vi "Persistence.vi"() -> ()   [LabVIEW 2022 SP3]
uses:
  ColorSelection.ctl
  d94e0766-a9f8-4b91-b199-a4dd9911b6b9.vi
  <vilib>/measure/NI_MABase.lvlib
  ed4c178f-8d92-4741-ab18-05d4051c7f8b.vi
panel:
  out "2nd Palette":u32[](array[colorbox])=[16711680, 16715535, 16719390, 16723245, 16727100, 16730955, 16734810, 16738665, 16742520, 16746375, 16750230, 16754085, 16757940, 16761795, 16765650, 16769505, 16773360]
  in  "2ndColor":T1
  in  "Buffer Depth IN":i32=17
  in  "1stColor":T1=enum."Green"
  out "1st Palette":u32[](array[colorbox])=[65280, 1048335, 2031390, 3014445, 3997500, 4980555, 5963610, 6946665, 7929720, 8912775, 9895830, 10878885, 11861940, 12844995, 13828050, 14811105, 15794160]
  in  "Color 2":T1
  in  "Color 1":T1=enum."Green"
  out "Palette 2":u32[](array[colorbox])=[16711680, 16715535, 16719390, 16723245, 16727100, 16730955, 16734810, 16738665, 16742520, 16746375, 16750230, 16754085, 16757940, 16761795, 16765650, 16769505, 16773360]
  in  "Signal Type 2":enum16{"Sine", "Gauss", "Sine + Gauss"}(ring)=enum."Sine + Gauss"
  out "Buffer Depth 2":i32=17
  out "Buffer Depth 1":i32=17
  in  "Combine signals to Signal 2":enum16{"None", "Add 1 and 2"}(ring)
  in  "Signal Type 1":enum16{"Sine", "Gauss", "Sine + Gauss"}(ring)=enum."Sine + Gauss"
  in  "frequency 2":dbl=3.0 format="%0.2p"
  in  "amplitude 2":dbl=0.75 format="%0.2p"
  in  "phase 2 [deg]":dbl=-2.0
  in  "sampling info 2":cluster{"Fs":dbl, "#s":dbl}={"Fs"=1000.0, "#s"=1000.0} {"Fs" format="%.2p"}
  out "Palette 1":u32[](array[colorbox])=[65280, 1048335, 2031390, 3014445, 3997500, 4980555, 5963610, 6946665, 7929720, 8912775, 9895830, 10878885, 11861940, 12844995, 13828050, 14811105, 15794160]
  in  "Persistence Depth":u32=17
  out "Combined Plots":waveform(dbl)[](graph)=[{"t0"=timestamp(0 s since 1904-01-01), "dt"=0.001, "Y"=array[1000 elements]}, {"t0"=timestamp(0 s since 1904-01-01), "dt"=0.001, "Y"=array[1000 elements]}, {"t0"=timestamp(0 s since 1904-01-01), "dt"=0.001, "Y"=array[1000 elements]}, {"t0"=timestamp(0 s since 1904-01-01), "dt"=0.001, "Y"=array[1000 elements]}, {"t0"=timestamp(0 s since 1904-01-01), "dt"=0.001, "Y"=array[1000 elements]}, {"t0"=timestamp(0 s since 1904-01-01), "dt"=0.001, "Y"=array[1000 elements]}, {"t0"=timestamp(0 s since 1904-01-01), "dt"=0.001, "Y"=array[1000 elements]}, {"t0"=timestamp(0 s since 1904-01-01), "dt"=0.001, "Y"=array[1000 elements]}, {"t0"=timestamp(0 s since 1904-01-01), "dt"=0.001, "Y"=array[1000 elements]}, {"t0"=timestamp(0 s since 1904-01-01), "dt"=0.001, "Y"=array[1000 elements]}, {"t0"=timestamp(0 s since 1904-01-01), "dt"=0.001, "Y"=array[1000 elements]}, {"t0"=timestamp(0 s since 1904-01-01), "dt"=0.001, "Y"=array[1000 elements]}, {"t0"=timestamp(0 s since 1904-01-01), "dt"=0.001, "Y"=array[1000 elements]}, {"t0"=timestamp(0 s since 1904-01-01), "dt"=0.001, "Y"=array[1000 elements]}, {"t0"=timestamp(0 s since 1904-01-01), "dt"=0.001, "Y"=array[1000 elements]}, {"t0"=timestamp(0 s since 1904-01-01), "dt"=0.001, "Y"=array[1000 elements]}, {"t0"=timestamp(0 s since 1904-01-01), "dt"=0.001, "Y"=array[1000 elements]}, {"t0"=timestamp(0 s since 1904-01-01), "dt"=0.001, "Y"=array[1000 elements]}, {"t0"=timestamp(0 s since 1904-01-01), "dt"=0.001, "Y"=array[1000 elements]}, {"t0"=timestamp(0 s since 1904-01-01), "dt"=0.001, "Y"=array[1000 elements]}, {"t0"=timestamp(0 s since 1904-01-01), "dt"=0.001, "Y"=array[1000 elements]}, {"t0"=timestamp(0 s since 1904-01-01), "dt"=0.001, "Y"=array[1000 elements]}, {"t0"=timestamp(0 s since 1904-01-01), "dt"=0.001, "Y"=array[1000 elements]}, {"t0"=timestamp(0 s since 1904-01-01), "dt"=0.001, "Y"=array[1000 elements]}, {"t0"=timestamp(0 s since 1904-01-01), "dt"=0.001, "Y"=array[1000 elements]}, {"t0"=timestamp(0 s since 1904-01-01), "dt"=0.001, "Y"=array[1000 elements]}, {"t0"=timestamp(0 s since 1904-01-01), "dt"=0.001, "Y"=array[1000 elements]}, {"t0"=timestamp(0 s since 1904-01-01), "dt"=0.001, "Y"=array[1000 elements]}, {"t0"=timestamp(0 s since 1904-01-01), "dt"=0.001, "Y"=array[1000 elements]}, {"t0"=timestamp(0 s since 1904-01-01), "dt"=0.001, "Y"=array[1000 elements]}, {"t0"=timestamp(0 s since 1904-01-01), "dt"=0.001, "Y"=array[1000 elements]}, {"t0"=timestamp(0 s since 1904-01-01), "dt"=0.001, "Y"=array[1000 elements]}, {"t0"=timestamp(0 s since 1904-01-01), "dt"=0.001, "Y"=array[1000 elements]}, {"t0"=timestamp(0 s since 1904-01-01), "dt"=0.001, "Y"=array[1000 elements]}]
  in  "frequency":dbl=10.0 format="%0.2p"
  in  "amplitude":dbl=1.0 format="%0.2p"
  in  "phase [deg]":dbl=3.0
  in  "sampling info":cluster{"Fs":dbl, "#s":dbl}={"Fs"=1000.0, "#s"=1000.0} {"Fs" format="%.2p"}
  in  "stop":bool
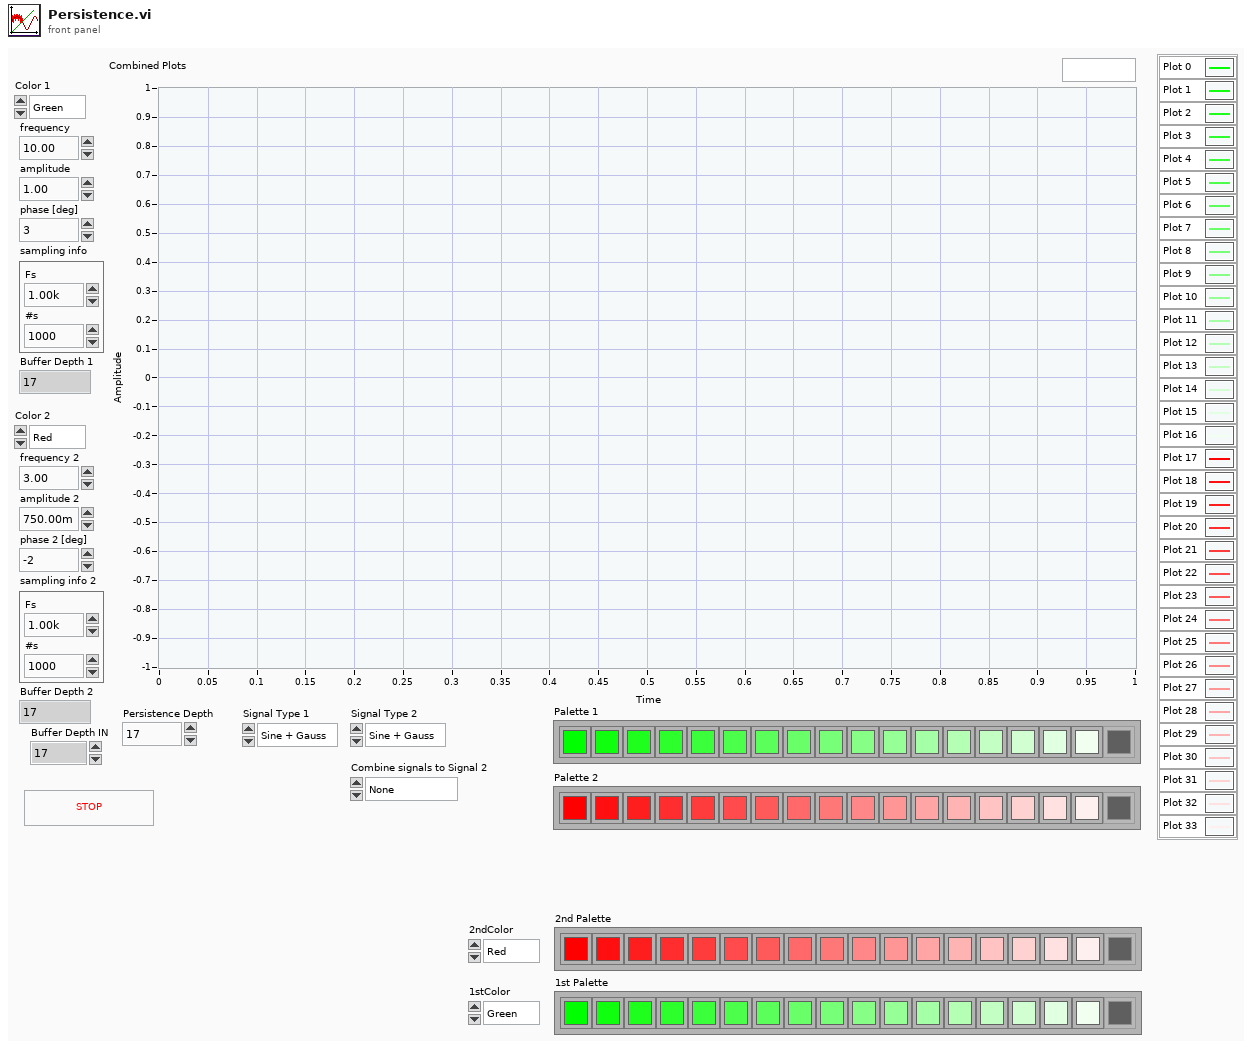
[diagram p1: front panel]
types:
  T1 = typedef "ColorSelection.ctl" = enum16{"Red", "Green", "Blue", "Yellow", "Magenta", "Cyan", "White", "Black"}
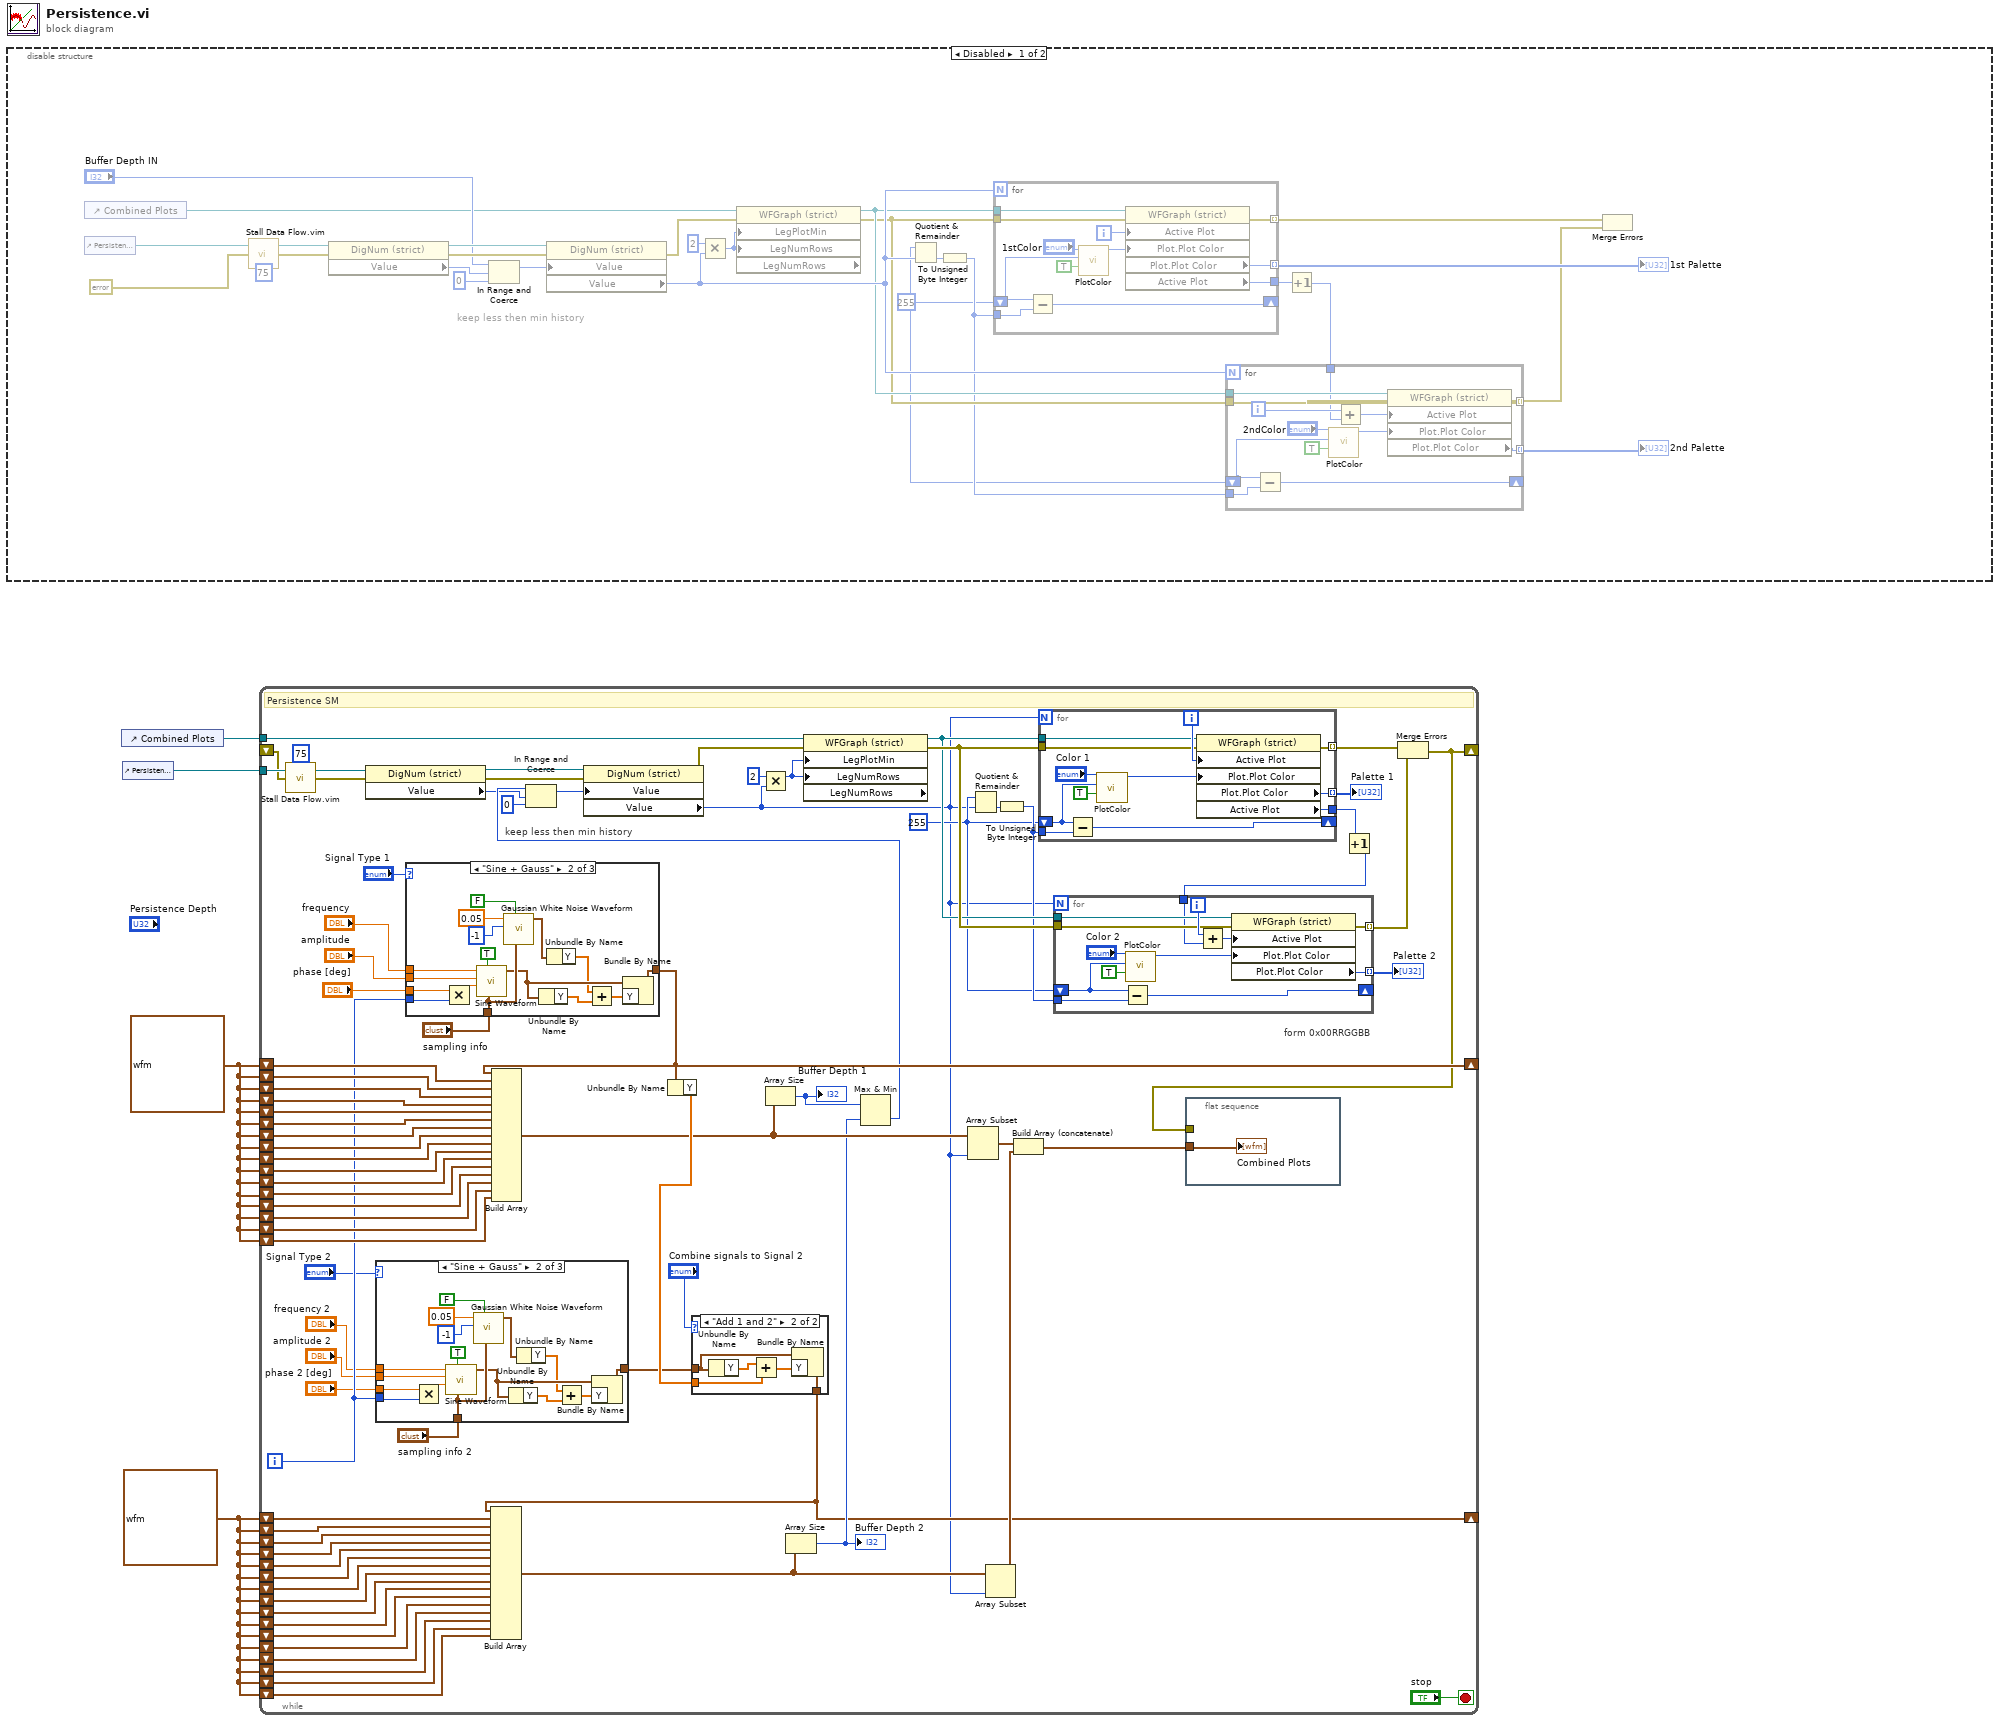
[diagram p0: block diagram]
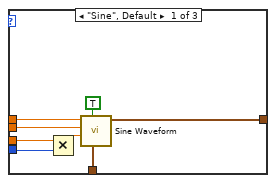
[diagram p3: hidden frame]
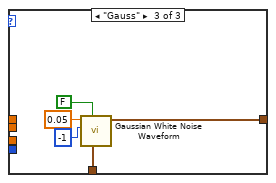
[diagram p4: hidden frame]
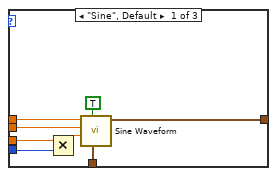
[diagram p6: hidden frame]
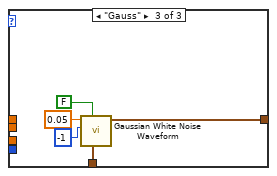
[diagram p7: hidden frame]
diagram:
  w4 = waveform(dbl) {"t0"=timestamp(0 s since 1904-01-01), "dt"=1.0, "Y"=[]} ("signal out")
  w3 = waveform(dbl) {"t0"=timestamp(0 s since 1904-01-01), "dt"=1.0, "Y"=[]} ("signal out")
  n1 = disable-structure shown="Disabled" {
    frame Disabled {
      w6 = u8 255
      # "keep less then min history"
      n2 = control-ref of="Combined Plots"() -> (w13:refnum<vi>)
      n3 = control-ref of="Persistence Depth"() -> (w16:refnum<vi>)
      n4 = call "Stall Data Flow.vim"("value in"=errorcluster {"status"=FALSE, "code"=0, "source"=""} ("error out"), "milliseconds to wait"=u32 75) -> ("value out"=w15:errorcluster)  [unwired: 1 out]
      n5 = property class="DigNum (strict)"(reference=w16, error in=w15) -> (reference out=w25:refnum<vi>, error out=w27:errorcluster, "Value"=w17:u32)
      n6 = In Range and Coerce(upper limit="Buffer Depth IN", x=w17, lower limit=u32 0) -> (coerced(x)=w26:u32)  [unwired: 1 out]
      n7 = property class="DigNum (strict)"(reference=w25, error in=w27, "Value"=w26) -> (error out=w28:errorcluster, "Value"=w12:u32)  [unwired: 1 out]
      n8 = Multiply(x=u32 2 ("y"), y=w12) -> (x*y=w22:u32)
      n9 = property on="Property Node" class="WFGraph (strict)" props=["LegPlotMin", "LegNumRows", "LegNumRows"](reference=w13, error in=w28, "LegPlotMin"=w22, "LegNumRows"=w22) -> (reference out=w11:refnum<vi>, error out=w10:errorcluster)  [unwired: 1 out]
      n10 = Quotient & Remainder(x=w6, y=w12) -> (floor(x/y)=w19:u32)  [unwired: 1 out]
      n11 = To Unsigned Byte Integer(number=w19) -> (unsigned 8bit integer=w7:u8)
      n12 = for {
        N: w12 -> [_]
        shift-right: [w52] -> _
        shift-left: w6 -> [w46]
        tunnel: w7 -> [w53]
        tunnel: w11 -> [w51]
        tunnel: w10 -> [w50]
        tunnel: [w49] -> w20 mode=indexing
        tunnel: [w48] -> w21
        tunnel: [w47] -> w29 mode=indexing
        i -> [w55]
        n13 = Subtract(x=w46, y=w53) -> (x-y=w52:u8)
        n14 = call "PlotColor.vi"("White Palette"=TRUE, "InputColorCode"=w46, "Color"="1stColor") -> ("Color"=w54:u32)  [unwired: 8 in]
        n15 = property on="Property Node" class="WFGraph (strict)"(reference=w51, error in=w50, "Active Plot"=w55, "Plot.Plot Color"=w54) -> (error out=w47:errorcluster, "Plot.Plot Color"=w49:u32, "Active Plot"=w48:u32)  [unwired: 1 out]
      }
      "1st Palette" <- w20
      n16 = Increment(x=w21) -> (x+1=w8:u32)
      n17 = for {
        N: w12 -> [_]
        shift-right: [w41] -> _
        shift-left: w6 -> [w37]
        tunnel: w7 -> [w42]
        tunnel: w11 -> [w40]
        tunnel: w10 -> [w39]
        tunnel: [w38] -> w9 mode=indexing
        tunnel: w8 -> [w32]
        tunnel: [w31] -> w5 mode=indexing
        i -> [w34]
        n18 = Subtract(x=w37, y=w42) -> (x-y=w41:u8)
        n19 = call "PlotColor.vi"("White Palette"=TRUE, "InputColorCode"=w37, "Color"="2ndColor") -> ("Color"=w43:u32)  [unwired: 8 in]
        n20 = Add(x=w34, y=w32) -> (x+y=w33:u32)
        n21 = property on="Property Node" class="WFGraph (strict)"(reference=w40, error in=w39, "Active Plot"=w33, "Plot.Plot Color"=w43) -> (error out=w38:errorcluster, "Plot.Plot Color"=w31:u32)  [unwired: 1 out]
      }
      "2nd Palette" <- w5
      n22 = Merge Errors(w29, w9) -> ()  [unwired: 1 out]
    }
    frame Enabled {
    }
  }
  n23 = control-ref of="Combined Plots"() -> (w2:refnum<vi>)
  n24 = control-ref of="Persistence Depth"() -> (w1:refnum<vi>)
  n25 = while {
    shift-right: [w97] -> _
    shift-left: w3 -> [w127]
    shift-left: w3 -> [w136]
    shift-left: w3 -> [w135]
    shift-left: w3 -> [w134]
    shift-left: w3 -> [w133]
    shift-left: w3 -> [w132]
    shift-left: w3 -> [w131]
    shift-left: w3 -> [w130]
    shift-left: w3 -> [w129]
    shift-left: w3 -> [w128]
    shift-left: w3 -> [w126]
    shift-left: w3 -> [w125]
    shift-right: [w78] -> _
    shift-left: w4 -> [w121]
    shift-left: w4 -> [w120]
    shift-left: w4 -> [w119]
    shift-left: w4 -> [w118]
    shift-left: w4 -> [w117]
    shift-left: w4 -> [w116]
    shift-left: w4 -> [w115]
    shift-left: w4 -> [w114]
    shift-left: w4 -> [w113]
    shift-left: w4 -> [w112]
    shift-left: w4 -> [w111]
    shift-left: w4 -> [w110]
    shift-left: w4 -> [w109]
    shift-left: w4 -> [w108]
    shift-left: w3 -> [w94]
    shift-left: w3 -> [w93]
    shift-left: w3 -> [w92]
    shift-left: w4 -> [w81]
    shift-left: w4 -> [w80]
    shift-left: w3 -> [w79]
    tunnel: w2 -> [w77]
    tunnel: w1 -> [w76]
    shift-right: [w56] -> _
    shift-left: _ -> [w59]
    i -> [w67]
    stop <- "stop" stop-if-true
    w103 = u8 255
    # "keep less then min history"
    # "form 0x00RRGGBB"
    # "Persistence SM"
    n26 = call "Stall Data Flow.vim"("value in"=w59, "milliseconds to wait"=u32 75) -> ("value out"=w58:errorcluster)  [unwired: 1 out]
    n27 = property class="DigNum (strict)"(reference=w76, error in=w58) -> (reference out=w83:refnum<vi>, error out=w75:errorcluster, "Value"=w84:u32)
    n28 = case shown="\"Sine + Gauss\"" "Signal Type 2" {
      tunnel: "sampling info 2" -> [w141 w154 w164]
      tunnel: w67 -> [w145 w161 _]
      tunnel: [w140 w150 w165] -> w69
      tunnel: "phase 2 [deg]" -> [w144 w160 _]
      tunnel: "amplitude 2" -> [w143 w159 _]
      tunnel: "frequency 2" -> [w142 w158 _]
      frame "Sine", Default {
        n29 = Multiply(x=w144, y=w145) -> (x*y=w146:dbl)
        n30 = call <vilib>:"Sine Waveform.vi"("sampling info"=w141, "reset signal"=TRUE, "phase"=w146, "amplitude"=w143, "frequency"=w142) -> ("signal out"=w140:waveform(dbl))  [unwired: 5 in, 1 out]
      }
      frame "Sine + Gauss" {
        n31 = Multiply(x=w160, y=w161) -> (x*y=w162:dbl)
        n32 = call <vilib>:"Sine Waveform.vi"("sampling info"=w154, "reset signal"=TRUE, "phase"=w162, "amplitude"=w159, "frequency"=w158) -> ("signal out"=w151:waveform(dbl))  [unwired: 5 in, 1 out]
        n33 = call <vilib>:"Gaussian White Noise Waveform.vi"("sampling info"=w154, "reset signal"=FALSE, "seed"=-1, "standard deviation"=0.05) -> ("signal out"=w149:waveform(dbl))  [unwired: 6 in, 1 out]
        n34 = Unbundle By Name(w151) -> ("Y"=w153:dbl[])
        n35 = Unbundle By Name(w149) -> ("Y"=w148:dbl[])
        n36 = Add(x=w148, y=w153) -> (x+y=w152:dbl[])
        n37 = Bundle By Name(cluster=w151, "Y"=w152) -> (w150:waveform(dbl))
      }
      frame "Gauss" {
        n38 = call <vilib>:"Gaussian White Noise Waveform.vi"("sampling info"=w164, "reset signal"=FALSE, "seed"=-1, "standard deviation"=0.05) -> ("signal out"=w165:waveform(dbl))  [unwired: 6 in, 1 out]
      }
    }
    n39 = case shown="\"Sine + Gauss\"" "Signal Type 1" {
      tunnel: "sampling info" -> [w176 w189 w199]
      tunnel: w67 -> [w180 w196 _]
      tunnel: [w175 w185 w200] -> w97
      tunnel: "phase [deg]" -> [w179 w195 _]
      tunnel: "amplitude" -> [w178 w194 _]
      tunnel: "frequency" -> [w177 w193 _]
      frame "Sine", Default {
        n40 = Multiply(x=w179, y=w180) -> (x*y=w181:dbl)
        n41 = call <vilib>:"Sine Waveform.vi"("sampling info"=w176, "reset signal"=TRUE, "phase"=w181, "amplitude"=w178, "frequency"=w177) -> ("signal out"=w175:waveform(dbl))  [unwired: 5 in, 1 out]
      }
      frame "Sine + Gauss" {
        n42 = Multiply(x=w195, y=w196) -> (x*y=w197:dbl)
        n43 = call <vilib>:"Sine Waveform.vi"("sampling info"=w189, "reset signal"=TRUE, "phase"=w197, "amplitude"=w194, "frequency"=w193) -> ("signal out"=w186:waveform(dbl))  [unwired: 5 in, 1 out]
        n44 = call <vilib>:"Gaussian White Noise Waveform.vi"("sampling info"=w189, "reset signal"=FALSE, "seed"=-1, "standard deviation"=0.05) -> ("signal out"=w184:waveform(dbl))  [unwired: 6 in, 1 out]
        n45 = Unbundle By Name(w186) -> ("Y"=w188:dbl[])
        n46 = Unbundle By Name(w184) -> ("Y"=w183:dbl[])
        n47 = Add(x=w183, y=w188) -> (x+y=w187:dbl[])
        n48 = Bundle By Name(cluster=w186, "Y"=w187) -> (w185:waveform(dbl))
      }
      frame "Gauss" {
        n49 = call <vilib>:"Gaussian White Noise Waveform.vi"("sampling info"=w199, "reset signal"=FALSE, "seed"=-1, "standard deviation"=0.05) -> ("signal out"=w200:waveform(dbl))  [unwired: 6 in, 1 out]
      }
    }
    n50 = Build Array(w97, w127, w136, w135, w134, w133, w132, w131, w130, w129, w128, w126, w125, w94, w93, w92, w79) -> (w91:waveform(dbl)[])
    n51 = Unbundle By Name(w97) -> ("Y"=w96:dbl[])
    n52 = case shown="\"Add 1 and 2\"" "Combine signals to Signal 2" {
      tunnel: w69 -> [w169 w173]
      tunnel: [w169 w172] -> w78
      tunnel: w96 -> [_ w170]
      frame "None", Default {
      }
      frame "Add 1 and 2" {
        n53 = Unbundle By Name(w173) -> ("Y"=w174:dbl[])
        n54 = Add(x=w174, y=w170) -> (x+y=w171:dbl[])
        n55 = Bundle By Name(cluster=w173, "Y"=w171) -> (w172:waveform(dbl))
      }
    }
    n56 = Build Array(w78, w121, w120, w119, w118, w117, w116, w115, w114, w113, w112, w111, w110, w109, w108, w81, w80) -> (w89:waveform(dbl)[])
    n57 = Array Size(array=w91) -> (size(s)=w88:i32)
    "Buffer Depth 1" <- w88
    n58 = Array Size(array=w89) -> (size(s)=w87:i32)
    "Buffer Depth 2" <- w87
    n59 = Max & Min(x=w88, y=w87) -> (min(x,y)=w86:i32)  [unwired: 1 out]
    n60 = In Range and Coerce(upper limit=w86, x=w84, lower limit=u32 0) -> (coerced(x)=w82:u32)  [unwired: 1 out]
    n61 = property class="DigNum (strict)"(reference=w83, error in=w75, "Value"=w82) -> (error out=w74:errorcluster, "Value"=w73:u32)  [unwired: 1 out]
    n62 = Multiply(x=u32 2 ("y"), y=w73) -> (x*y=w101:u32)
    n63 = property on="Property Node" class="WFGraph (strict)" props=["LegPlotMin", "LegNumRows", "LegNumRows"](reference=w77, error in=w74, "LegPlotMin"=w101, "LegNumRows"=w101) -> (reference out=w105:refnum<vi>, error out=w106:errorcluster)  [unwired: 1 out]
    n64 = Array Subset(array=w91, length=w73) -> (w123:waveform(dbl)[])  [unwired: 1 in]
    n65 = Quotient & Remainder(x=w103, y=w73) -> (floor(x/y)=w124:u32)  [unwired: 1 out]
    n66 = Array Subset(array=w89, length=w73) -> (w90:waveform(dbl)[])  [unwired: 1 in]
    n67 = To Unsigned Byte Integer(number=w124) -> (unsigned 8bit integer=w104:u8)
    n68 = Build Array (concatenate)(w123, w90) -> (w107:waveform(dbl)[])
    n69 = for {
      N: w73 -> [_]
      shift-right: [w225] -> _
      shift-left: w103 -> [w219]
      tunnel: w104 -> [w226]
      tunnel: w105 -> [w224]
      tunnel: w106 -> [w223]
      tunnel: [w222] -> w122 mode=indexing
      tunnel: [w221] -> w102
      tunnel: [w220] -> w61 mode=indexing
      i -> [w228]
      n70 = Subtract(x=w219, y=w226) -> (x-y=w225:u8)
      n71 = call "PlotColor.vi"("White Palette"=TRUE, "InputColorCode"=w219, "Color"="Color 1") -> ("Color"=w227:u32)  [unwired: 8 in]
      n72 = property on="Property Node" class="WFGraph (strict)"(reference=w224, error in=w223, "Active Plot"=w228, "Plot.Plot Color"=w227) -> (error out=w220:errorcluster, "Plot.Plot Color"=w222:u32, "Active Plot"=w221:u32)  [unwired: 1 out]
    }
    "Palette 1" <- w122
    n73 = flat-sequence {
      tunnel: w107 -> [w139]
      tunnel: w56 -> [_]
      frame #0 {
        "Combined Plots" <- w139
      }
    }
    n74 = Increment(x=w102) -> (x+1=w99:u32)
    n75 = for {
      N: w73 -> [_]
      shift-right: [w214] -> _
      shift-left: w103 -> [w205]
      tunnel: w104 -> [w215]
      tunnel: w105 -> [w213]
      tunnel: w106 -> [w212]
      tunnel: [w211] -> w62 mode=indexing
      tunnel: w99 -> [w209]
      tunnel: [w208] -> w60 mode=indexing
      i -> [w216]
      n76 = Subtract(x=w205, y=w215) -> (x-y=w214:u8)
      n77 = call "PlotColor.vi"("White Palette"=TRUE, "InputColorCode"=w205, "Color"="Color 2") -> ("Color"=w204:u32)  [unwired: 8 in]
      n78 = Add(x=w216, y=w209) -> (x+y=w210:u32)
      n79 = property on="Property Node" class="WFGraph (strict)"(reference=w213, error in=w212, "Active Plot"=w210, "Plot.Plot Color"=w204) -> (error out=w208:errorcluster, "Plot.Plot Color"=w211:u32)  [unwired: 1 out]
    }
    "Palette 2" <- w62
    n80 = Merge Errors(w61, w60) -> (w56:errorcluster)
  }
